vi "CH_LM Config Trigger External.vi"(0 "Meter Index":i32, 2 "Trigger Slope (pos.)":bool=TRUE, 3 "Trigger Delay (0µs)":dbl format="%#.3g", 5 "error in (no error)":errorcluster, 7 "Timeout / ms (3000)":i32=3000, 8 "Action (query)":bool, 9 "Lock Timeout / ms (1000)":i32=1000) -> (11 "Lock timed out":bool, 14 "Meter Index":i32, 16 "Trigger Slope":bool, 17 "Trigger Delay / µs":dbl format="%#.3g", 19 "error out":errorcluster)   [LabVIEW 2012, in "CH_LM.lvlib"]
doc: "This command will set/query the external trigger edge and delay time. \n\n<B>Note:</B> To be used with External Trigger Source."
uses:
  CH_LM.lvlib
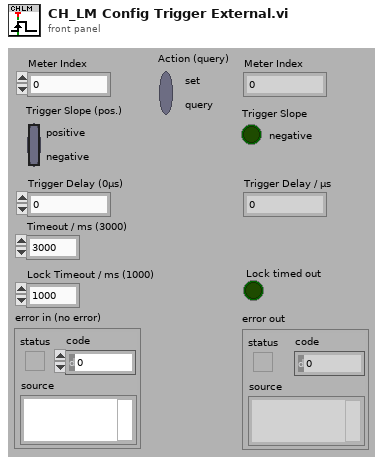
[diagram p1: front panel]
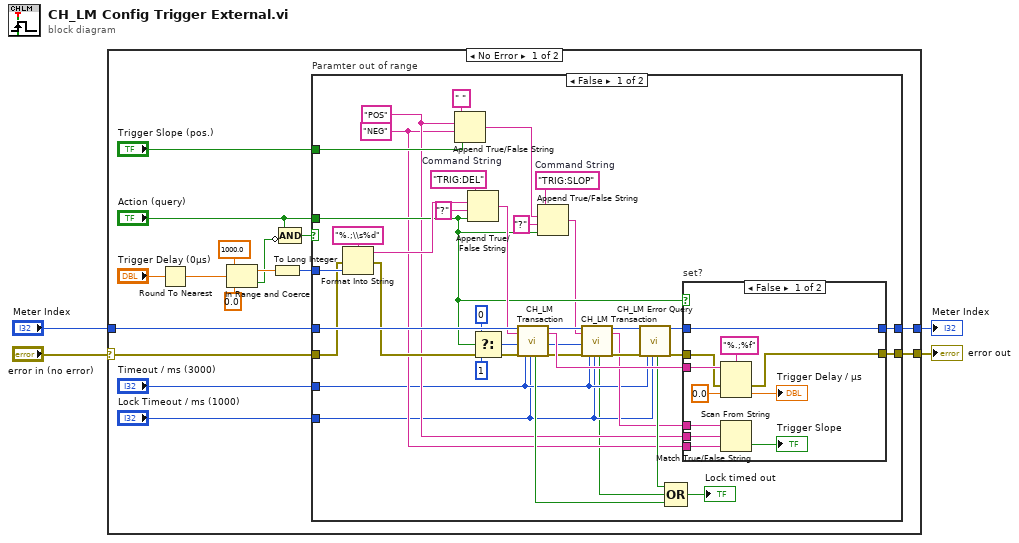
[diagram p0: block diagram]
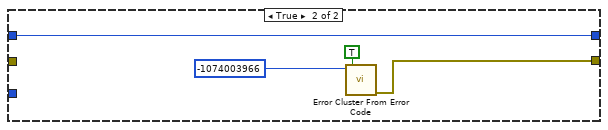
[diagram p3: hidden frame]
diagram:
  n1 = case shown="No Error" "error in (no error)" {
    selector: "error in (no error)" -> [w20 w76]
    tunnel: [w18 w76] -> w4
    tunnel: "Meter Index" -> [w19 w75]
    tunnel: [w17 w75] -> w1
    frame No Error {
      n2 = Round To Nearest(number="Trigger Delay (0µs)") -> (nearest integer value=w7:dbl)
      n3 = In Range and Coerce(upper limit=1000.0, x=w7, lower limit=0.0) -> (coerced(x)=w13:dbl, In Range?=w10:bool)
      n4 = To Long Integer(number=w13) -> (32bit integer=w6:i32)
      n5 = Compound Arithmetic op=AND("Action (query)", invert w10) -> (w8:bool)
      n6 = case "Paramter out of range" shown="False" w8 {
        tunnel: w20 -> [w42 _]
        tunnel: w19 -> [w57 w74]
        tunnel: [w54 w72] -> w18
        tunnel: [w49 w74] -> w17
        tunnel: "Timeout / ms (3000)" -> [w23 _]
        tunnel: "Lock Timeout / ms (1000)" -> [w22 _]
        tunnel: w6 -> [w43 _]
        tunnel: "Action (query)" -> [w32 _]
        tunnel: "Trigger Slope (pos.)" -> [w28 _]
        frame False {
          w24 = "NEG" ("false string")
          w25 = "POS" ("true string")
          w33 = "TRIG:SLOP"  # Command String
          w56 = "TRIG:DEL"  # Command String
          n7 = Format Into String(format string="%.;\\s%d", error in=w42, w43) -> (resulting string=w39:string, error out=w41:errorcluster)  [unwired: 1 in]
          n8 = Append True/False String(1:w28, 2:w24, 3:w25, 4:" " ("string (\"\")")) -> (0:w30:string)
          n9 = Append True/False String(1:w32, 2:"?" ("true string"), 3:w39, 4:w56) -> (0:w40:string)
          n10 = Select(t=0, s=w32, f=1 ("NofStrings (-1:all)")) -> (s? t:f=w27:i32)
          n11 = call "CH_LM Transaction.vi"("Meter Index"=w57, "Command String"=w40, "NofStrings (-1:all)"=w27, "error in (no error)"=w41, "Timeout / ms (3000)"=w23, "Lock Timeout / ms (1000)"=w22) -> ("Lock timed out"=w45:bool, "Meter Index"=w38:i32, "Response"=w55:string, "error out"=w37:errorcluster)  [unwired: 10 out]
          n12 = Append True/False String(1:w32, 2:"?" ("true string"), 3:w30, 4:w33) -> (0:w29:string)
          n13 = call "CH_LM Transaction.vi"("Meter Index"=w38, "Command String"=w29, "NofStrings (-1:all)"=w27, "error in (no error)"=w37, "Timeout / ms (3000)"=w23, "Lock Timeout / ms (1000)"=w22) -> ("Lock timed out"=w21:bool, "Meter Index"=w36:i32, "Response"=w26:string, "error out"=w35:errorcluster)  [unwired: 10 out]
          n14 = call "CH_LM Error Query.vi"("Meter Index"=w36, "error in (no error)"=w35, "Timeout / ms (3000)"=w23, "Lock Timeout / ms (1000)"=w22) -> ("Lock timed out"=w46:bool, "Meter Index"=w48:i32, "error out"=w47:errorcluster)  [unwired: 13 out]
          n15 = Compound Arithmetic op=OR(w46, w21, w45) -> (→"Lock timed out":bool)
          n16 = case "set?" shown="False" w32 {
            tunnel: w55 -> [w68 _]
            tunnel: w47 -> [w67 w70]
            tunnel: [w66 w70] -> w54
            tunnel: w48 -> [w63 w69]
            tunnel: [w63 w69] -> w49
            tunnel: w26 -> [w61 _]
            tunnel: w25 -> [w60 _]
            tunnel: w24 -> [w59 _]
            frame False {
              n17 = Scan From String(format string="%.;%f", input string=w68, error in=w67, default 1=0.0 ("default value 1")) -> (error out=w66:errorcluster, output 1=→"Trigger Delay / µs":dbl)  [unwired: 1 in, 2 out]
              n18 = Match True/False String(2:w59, 3:w60, 4:w61) -> (0:→"Trigger Slope":bool)  [unwired: 1 out]
            }
            frame True {
            }
          }
        }
        frame True {
          n19 = call <vilib>:"Error Cluster From Error Code.vi"("show call chain? (False)"=TRUE, "error code (0)"=-1074003966) -> ("error out"=w72:errorcluster)  [unwired: 1 in, 6 out]
        }
      }
    }
    frame Error {
    }
  }
  "error out" <- w4
  "Meter Index" <- w1
